vi "Read Users From File.vi"(8 "Error in":errorcluster caption="Error in (no error)") -> (0 "Error out":errorcluster, 3 "Array":T1[](array[typedef]))   [LabVIEW 2020]
uses:
  Typedef/User-Info.ctl
  Typedef/User-Role.ctl
  0a74098a-8fda-4e50-8bcc-1f710fccc8a0.vi
  <userlib>/NEVSTOP-Programming-Palette/Configuration/ClusterCfgTable/Parse CfgTable(with DataName).vi
  <userlib>/NEVSTOP-Programming-Palette/Configuration/Ini/ini_configuration_nevstop.lvlib
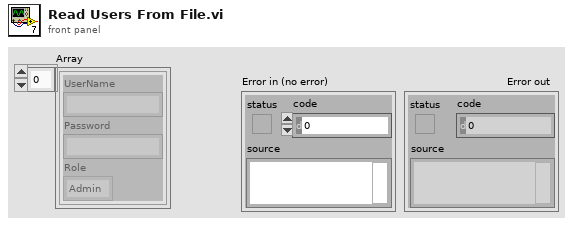
[diagram p1: front panel]
types:
  T1 = typedef "User-Info.ctl" = cluster{"UserName":string, "Password":string, "Role":T2}
  T2 = typedef "User-Role.ctl" = enum16{"Admin", "Engineer", "Operator"}
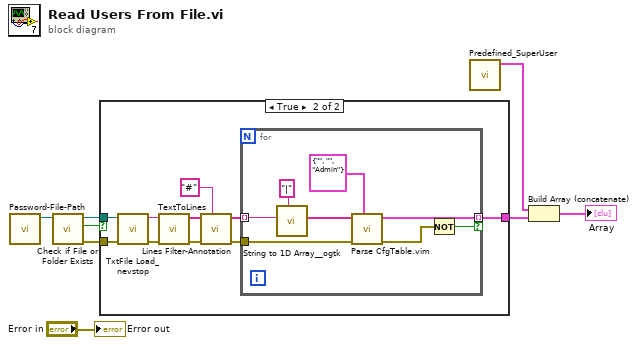
[diagram p0: block diagram]
diagram:
  n1 = call "Password-File-Path.vi"() -> ("Matched Config File"=w2:path)  [unwired: 11 in]
  n2 = call <vilib>:"Check if File or Folder Exists.vi"("path"=w2) -> ("error out"=w4:errorcluster, "file or folder exists?"=w6:bool, "dup path"=w3:path)  [unwired: 8 in]
  n3 = case shown="True" w6 {
    tunnel: w3 -> [_ w12]
    tunnel: w4 -> [_ w11]
    tunnel: [_ w10] -> w5
    frame False {
    }
    frame True {
      n4 = call <userlib>:"TxtFile Load_nevstop.vi"("error in (no error)"=w11, "Path"=w12) -> ("error out"=w18:errorcluster, "text"=w17:string)  [unwired: 8 in]
      n5 = call <userlib>:"TextToLines.vi"("error in (no error)"=w18, "string"=w17) -> ("error out"=w16:errorcluster, "Lines"=w15:string[])  [unwired: 8 in]
      n6 = call <userlib>:"Lines Filter-Annotation.vi"("Annotation Seperator(#)"="#", "error in (no error)"=w16, "Lines"=w15) -> ("error out"=w13:errorcluster, "Config Text List"=w14:string[])  [unwired: 7 in]
      n7 = for {
        tunnel: w14 -> [w26] mode=indexing
        tunnel: w13 -> [w25]
        tunnel: [w21] -> w10 mode=indexing if=w19
        n8 = call <userlib>:"String to 1D Array__ogtk.vi"("delimiter (Tab)"="|", "string"=w26) -> ("Array of Strings"=w24:string[])  [unwired: 9 in]
        n9 = call "Parse CfgTable.vim"("Cluster Configuration Typedef"=T1 {"UserName"="", "Password"="", "Role"=enum."Admin"}, "error in (no error)"=w25, "CfgTable Row"=w24) -> ("error out"=w20:errorcluster, "Cluster Configuration Out"=w21:T1)  [unwired: 7 in]
        n10 = Not(x=w20) -> (.not. x?=w19:bool)
      }
    }
  }
  n11 = call "Predefined_SuperUser.vi"() -> ("SuperUsers"=w7:T1[])  [unwired: 11 in]
  n12 = Build Array (concatenate)(w7, w5) -> (→"Array":T1[])
  "Error out" <- "Error in"
